vi "Create EUI Events.vi"(8 "error in (no error)":errorcluster, 11 "EUI Events in":refnum<class "EUI Events.lvclass">) -> (0 "error out":errorcluster, 3 "EUI Events out":refnum<class "EUI Events.lvclass">)   [LabVIEW 2016, in "EUI Events.lvclass"]
uses:
  EUI Events.lvclass
  Typedefs/MessageContainer.ctl
  EUI Events.lvclass/EUI Events.ctl
  Typedefs/M1M3SupportEUI_TypeDefs.lvlib
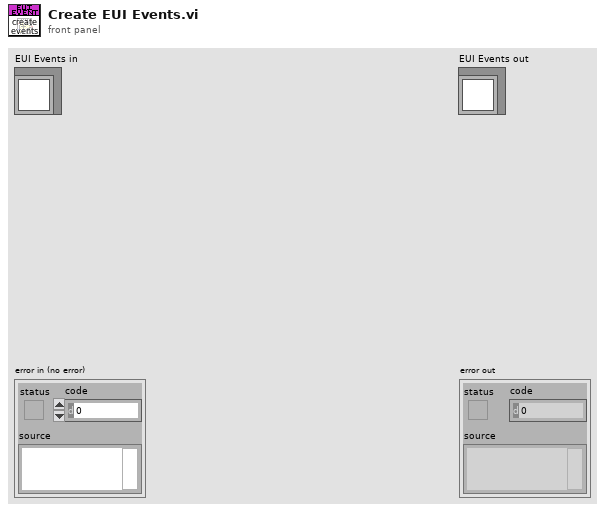
[diagram p1: front panel]
types:
  T1 = typedef "M1M3SupportEUI_TypeDefs.lvlib/MessageContainer.ctl" = cluster{"Message":string, "Time Stamp":timestamp, "Priority":enum16{"Message", "Warning", "Fault", ""}}
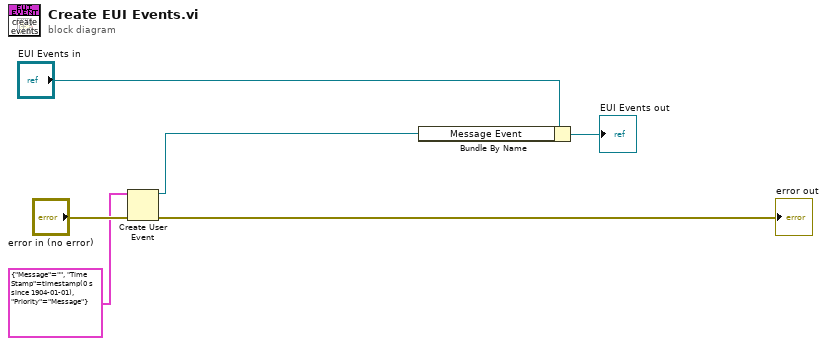
[diagram p0: block diagram]
diagram:
  n1 = Create User Event(user event datatype=T1 {"Message"="", "Time Stamp"=timestamp(0 s since 1904-01-01), "Priority"=enum."Message"} ("MessageCluster"), error in="error in (no error)") -> (user event=w2:refnum<user-event>, error out=→"error out":errorcluster)
  n2 = Bundle By Name(cluster="EUI Events in", "Message Event"=w2) -> (→"EUI Events out":refnum<class "EUI Events.lvclass">)
